vi "Read Velocity.vi"(8 "error in (no error)":errorcluster, 11 "Serial Controller in":refnum<class "Serial Controller.lvclass">) -> (0 "error out":errorcluster, 2 "Velocity":u16, 3 "Serial Controller out":refnum<class "Serial Controller.lvclass">)   [LabVIEW 2014, in "Serial Controller.lvclass"]
uses:
  Serial Controller.lvclass
  Serial Controller.lvclass/Serial Controller.ctl
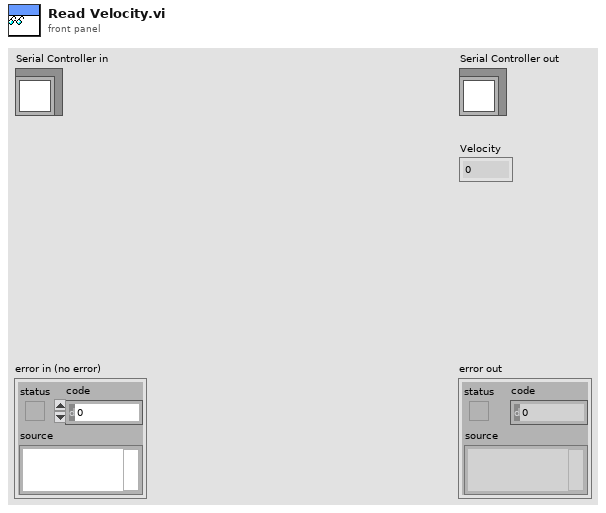
[diagram p1: front panel]
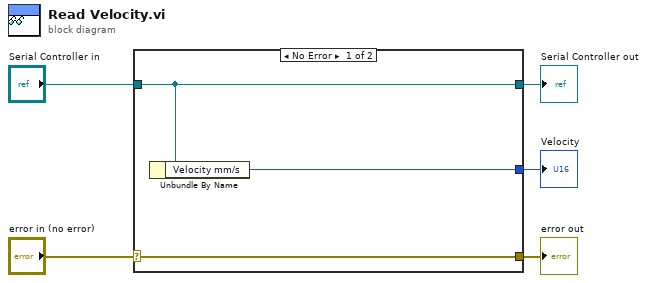
[diagram p0: block diagram]
diagram:
  n1 = case shown="No Error" "error in (no error)" {
    selector: "error in (no error)" -> [w8 w9]
    tunnel: [w8 w9] -> w4
    tunnel: [w7 w10] -> w2
    tunnel: "Serial Controller in" -> [w7 w10]
    tunnel: [w6 _] -> w1
    frame No Error {
      n2 = Unbundle By Name(w7) -> ("Velocity mm/s"=w6:u16)
    }
    frame Error {
    }
  }
  "error out" <- w4
  "Serial Controller out" <- w2
  "Velocity" <- w1
